vi "Host-Mac-Top.vi"() -> ()   [LabVIEW 2017]
uses:
  <vilib>/rvi/interface/nirviMethod/nirviMethod.xnode
  <vilib>/rvi/errors/niLvFpgaMergeErrorWithErrorCode.vi
  <vilib>/rvi/interface/nirviCloseFPGA/nirviCloseFPGA.xnode
  <vilib>/FPGAPlugInAG/Dynamic/niLvFpga_Close_Dynamic.vi
  MAC.Events.ctl
  <vilib>/rvi/interface/nirviOpenFPGA/nirviOpenFPGA.xnode
  <vilib>/FPGAPlugInAG/Dynamic/niLvFpga_ReadFifo_Dynamic.vi
  <vilib>/FPGAPlugInAG/Dynamic/niLvFpga_WriteFifo_Dynamic.vi
  FPGA Bitfiles/Fpga-Mac-Top.lvbitx
  FPGA/MAC/Fpga-Mac-Top.vi
  <vilib>/FPGAPlugInAG/PXIe-6592R/niLvFpga_Open_PXIe-6592R.vi
  <vilib>/rvi/interface/common/dynamic/niFpgaDynamicAddResources.vi
panel:
  in  "Ethernet II Params":T1={"Destination MAC"=[0, 2, 201, 85, 8, 68], "Source MAC"=[0, 1, 2, 3, 4, 5], "EtherType"=2048} {"Destination MAC" format="%.0x"; "Source MAC" format="%.02x"; "EtherType" format="%.0x"}
  in  "IPv4 Params":T2={"Destination IP"=[10, 0, 1, 100], "Source IP"=[10, 0, 1, 101], "Protocol"=17}
  in  "UDP Params":T3
  out "Status":string
  out "error out":errorcluster
  in  "Exit":bool
  in  "Transmit Packet":bool
  in  "Read Packet":bool
  out "RX Data":i32[](array[numeric])
  in  "error in":errorcluster
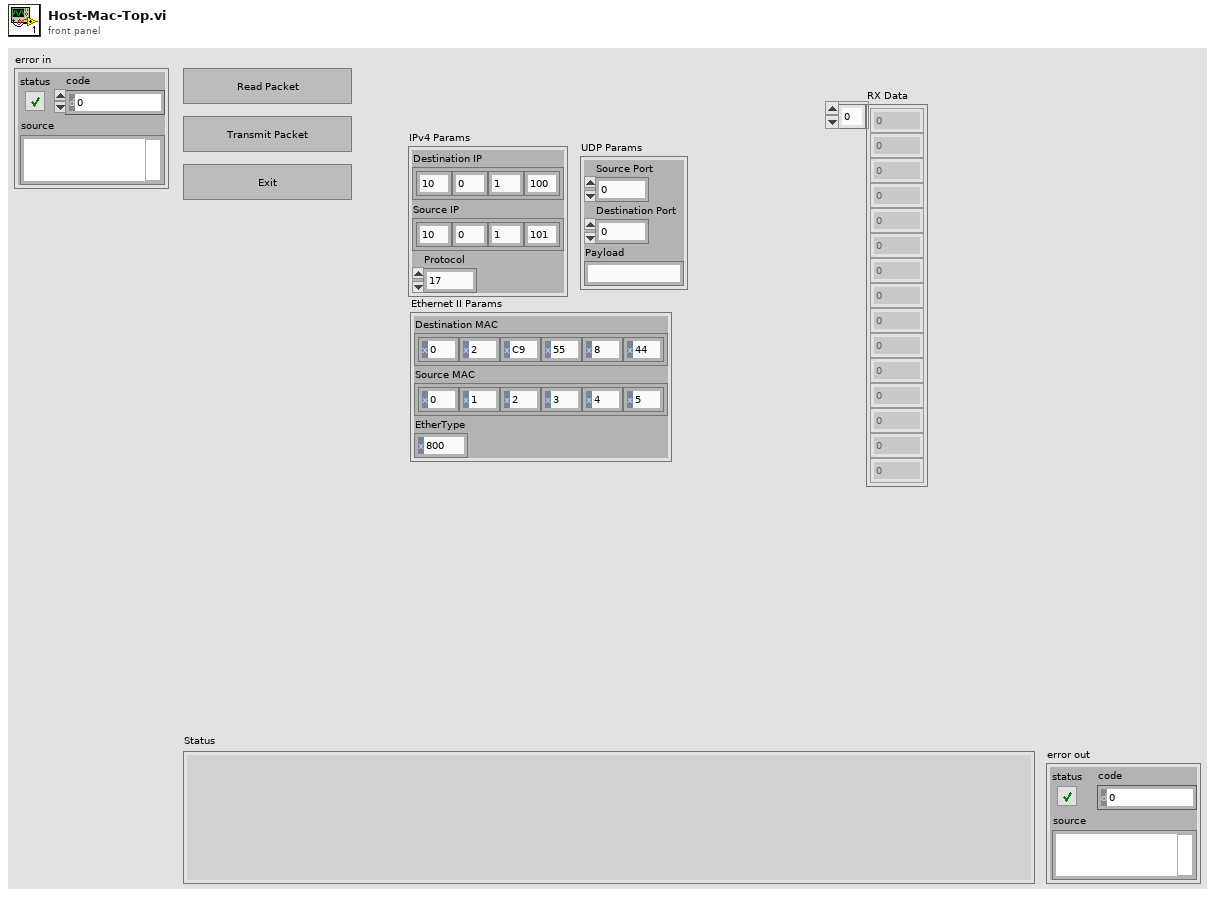
[diagram p1: front panel]
types:
  T1 = cluster{"Destination MAC":u8[], "Source MAC":u8[], "EtherType":u16}
  T2 = cluster{"Destination IP":u8[], "Source IP":u8[], "Protocol":u8}
  T3 = cluster{"Source Port":u16, "Destination Port":u16, "Payload":string}
  T4 = typedef "MAC.Events.ctl" = enum16{"Open FPGA", "Close FPGA", "Poll RX", "Transmit Packet"}
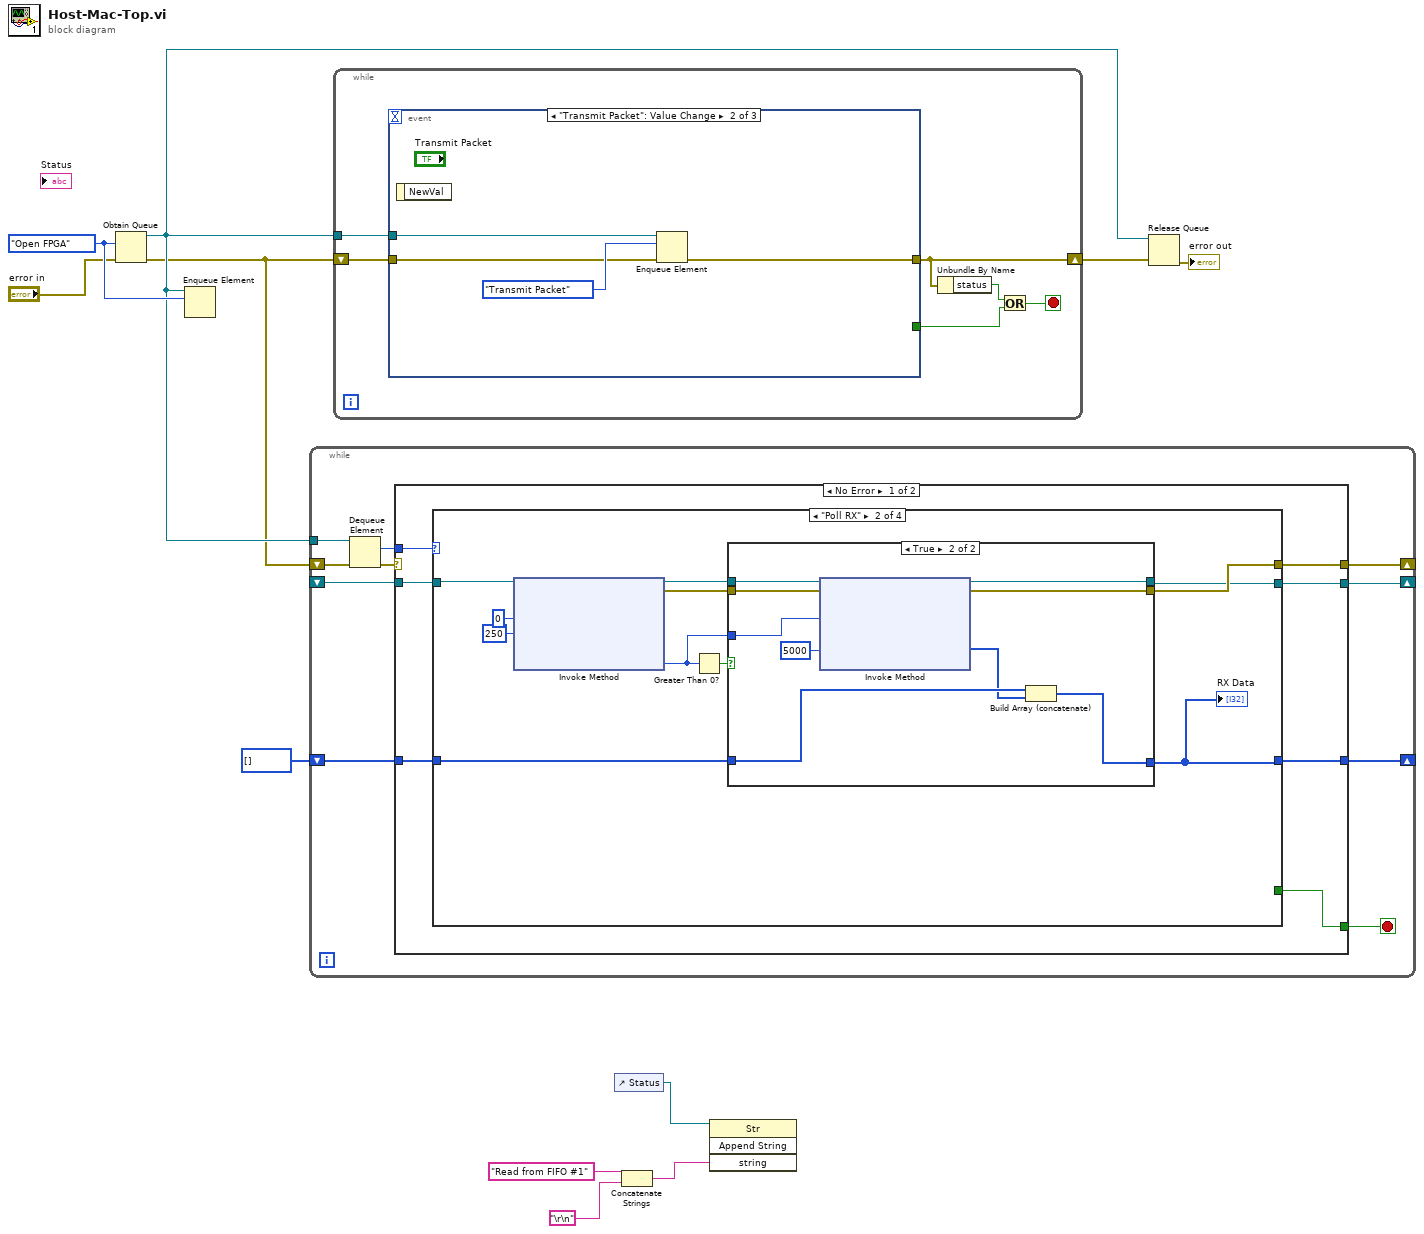
[diagram p0: block diagram]
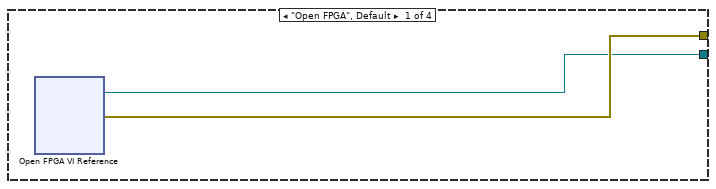
[diagram p2: hidden frame]
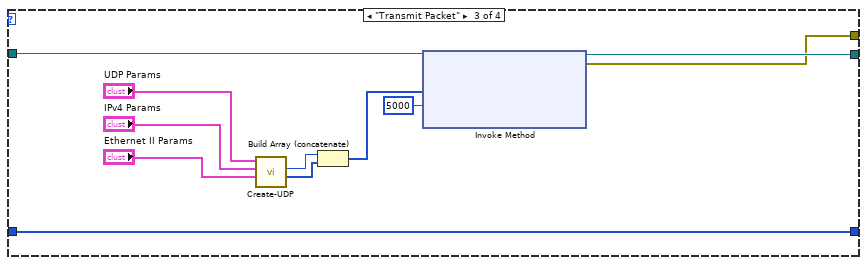
[diagram p4: hidden frame]
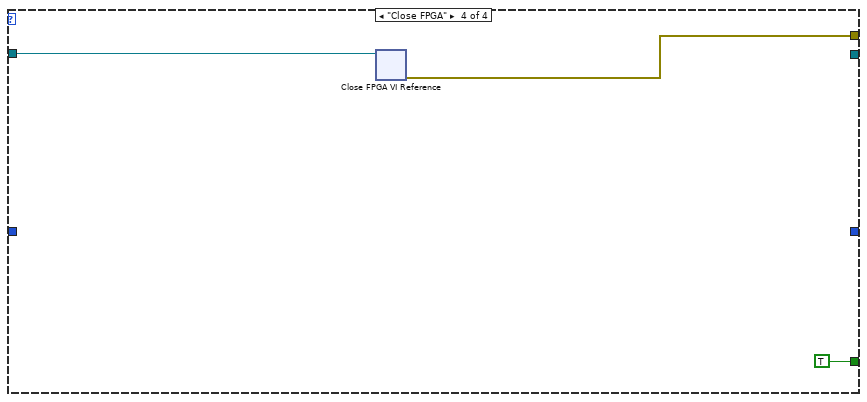
[diagram p5: hidden frame]
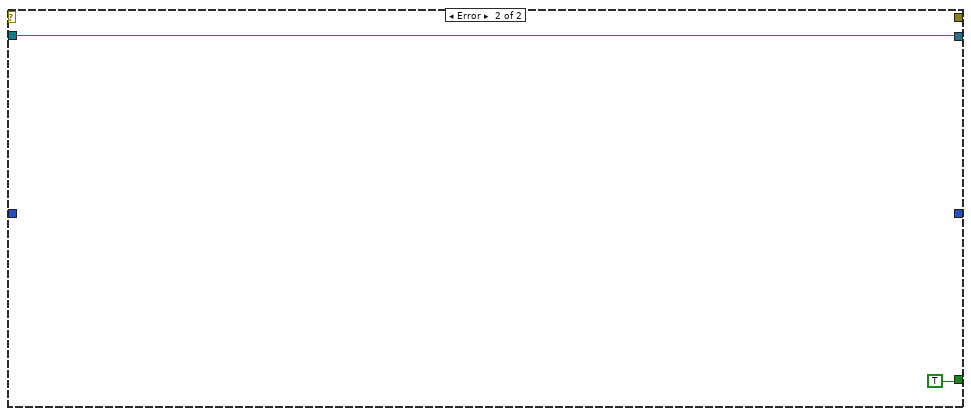
[diagram p6: hidden frame]
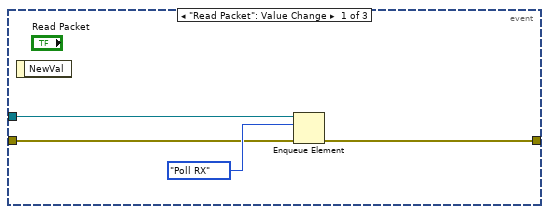
[diagram p7: hidden frame]
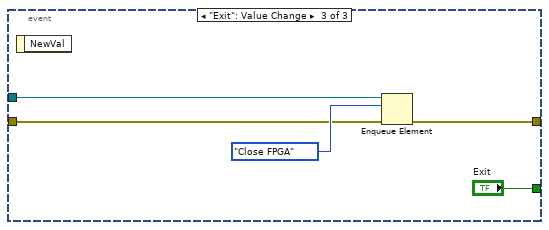
[diagram p8: hidden frame]
diagram:
  w11 = MAC.Events."Open FPGA"
  n1 = Obtain Queue(element data type=w11, error in (no error)="error in") -> (queue out=w8:refnum<queue>, error out=w6:errorcluster)  [unwired: 3 in, 1 out]
  n2 = Enqueue Element(queue=w8, element=w11) -> ()  [unwired: 2 in, 3 out]
  n3 = while {
    tunnel: w8 -> [w21]
    shift-right: [w16] -> _
    shift-left: w6 -> [w17]
    shift-right: [w15] -> _
    shift-left: _ -> [w14]
    shift-right: [w12] -> _
    shift-left: i32[] [] -> [w13]
    stop <- w18 stop-if-true
    n4 = Dequeue Element(queue=w21, error in (no error)=w17) -> (element=w19:T4, error out=w20:errorcluster)  [unwired: 1 in, 2 out]
    n5 = case shown="No Error" w20 {
      tunnel: w19 -> [w28 _]
      tunnel: [w27 TRUE] -> w18
      tunnel: [w26 _] -> w16
      tunnel: [w25 w68] -> w15
      tunnel: w14 -> [w24 w68]
      tunnel: w13 -> [w23 _]
      tunnel: [w22 _] -> w12
      frame No Error {
        n6 = case shown="\"Poll RX\"" w28 {
          tunnel: [_ _ _ TRUE] -> w27
          tunnel: [w30 w33 w54 w65] -> w26
          tunnel: [w29 w32 w55 _] -> w25
          tunnel: w24 -> [_ w34 w56 w66]
          tunnel: w23 -> [_ w35 w64 _]
          tunnel: [_ w31 w64 _] -> w22
          frame "Open FPGA", Default {
            n7 = xnode "Open FPGA VI Reference"() -> ("FPGA VI Reference Out"=w29:refnum<k20>, "error out"=w30:errorcluster)  [unwired: 2 in]
          }
          frame "Poll RX" {
            n8 = xnode "Invoke Method"("FPGA VI Reference In"=w34, "Number of Elements"=u32 0, "Timeout (ms)"=250) -> ("FPGA VI Reference Out"=w36:refnum<k20>, "error out"=w37:errorcluster, "Elements Remaining"=w38:u32)  [unwired: 1 in, 1 out]
            n9 = Greater Than 0?(x=w38) -> (x > 0?=w39:bool)
            n10 = case shown="True" w39 {
              tunnel: w38 -> [_ w53]
              tunnel: w37 -> [w43 w52]
              tunnel: w36 -> [w44 w51]
              tunnel: [w44 w49] -> w32
              tunnel: [w43 w48] -> w33
              tunnel: [w42 w45] -> w31
              tunnel: w35 -> [w42 w47]
              frame False {
              }
              frame True {
                n11 = xnode "Invoke Method"("FPGA VI Reference In"=w51, "error in"=w52, "Number of Elements"=w53, "Timeout (ms)"=5000) -> ("FPGA VI Reference Out"=w49:refnum<k20>, "error out"=w48:errorcluster, "Data"=w46:u8[])  [unwired: 1 out]
                n12 = Build Array (concatenate)(w47, w46) -> (w45:i32[])
              }
            }
            "RX Data" <- w31
          }
          frame "Transmit Packet" {
            n13 = call "Create-UDP.vi"("Ethernet II Params"="Ethernet II Params", "IPv4 Params"="IPv4 Params", "UDP Params"="UDP Params") -> ("Ethernet Frame\nU64"=w59:u64[], "Ethernet Frame\nsize"=w60:i32)  [unwired: 6 in, 1 out]
            n14 = Build Array (concatenate)(w60, w59) -> (w58:u64[])
            n15 = xnode "Invoke Method"("FPGA VI Reference In"=w56, "Data"=w58, "Timeout (ms)"=5000) -> ("FPGA VI Reference Out"=w55:refnum<k20>, "error out"=w54:errorcluster)  [unwired: 1 in, 1 out]
          }
          frame "Close FPGA" {
            n16 = xnode "Close FPGA VI Reference"("FPGA VI Reference In"=w66) -> ("error out"=w65:errorcluster)  [unwired: 1 in]
          }
        }
      }
      frame Error {
      }
    }
  }
  n17 = while {
    tunnel: w8 -> [w75]
    shift-right: [w70] -> w10
    shift-left: w6 -> [w71]
    stop <- w73 stop-if-true
    n18 = event shown="[1] \"Transmit Packet\": Value Change" {
      selector: _ -> [_ _ _]
      dyn-events: _ -> [_ _ _]
      timeout: _ -> [_ _ _]
      tunnel: w75 -> [w79 w82 w87]
      tunnel: [w77 w80 w86] -> w70
      tunnel: [_ _ "Exit"] -> w72
      tunnel: w71 -> [w76 w81 w84]
      event "Read Packet": Value Change {
        n19 = event-data() -> ()  [unwired: 1 in, 1 out]
        n20 = Enqueue Element(queue=w79, element=MAC.Events."Poll RX", error in (no error)=w76) -> (error out=w77:errorcluster)  [unwired: 1 in, 2 out]
      }
      event "Transmit Packet": Value Change {
        n21 = event-data() -> ()  [unwired: 1 in, 1 out]
        n22 = Enqueue Element(queue=w82, element=MAC.Events."Transmit Packet", error in (no error)=w81) -> (error out=w80:errorcluster)  [unwired: 1 in, 2 out]
      }
      event "Exit": Value Change {
        n23 = event-data() -> ()  [unwired: 1 in, 1 out]
        n24 = Enqueue Element(queue=w87, element=MAC.Events."Close FPGA", error in (no error)=w84) -> (error out=w86:errorcluster)  [unwired: 1 in, 2 out]
      }
    }
    n25 = Unbundle By Name(w70) -> ("status"=w74:bool)
    n26 = Or(x=w74, y=w72) -> (x .or. y?=w73:bool)
  }
  n27 = control-ref of="Status"() -> (w1:refnum<vi>)
  n28 = Concatenate Strings("Read from FIFO #1" ("string"), "\r\n") -> (w3:string)
  n29 = invoke class="Str" method="Append String"(reference=w1, "string"=w3) -> ()  [unwired: 2 in, 4 out]
  n30 = Release Queue(queue=w8, error in (no error)=w10) -> (error out=→"error out":errorcluster)  [unwired: 1 in, 2 out]
